vi "Read Fill.vi"(8 "error in (no error)":errorcluster, 11 "Rectangle in":refnum<class "Rectangle.lvclass">=refnum) -> (0 "error out":errorcluster, 2 "Fill":bool, 3 "Rectangle out":refnum<class "Rectangle.lvclass">)   [LabVIEW 2020]
uses:
  Rectangle.lvclass
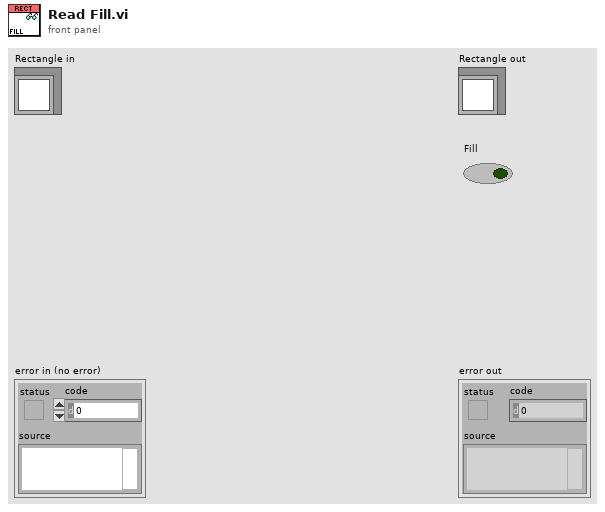
[diagram p1: front panel]
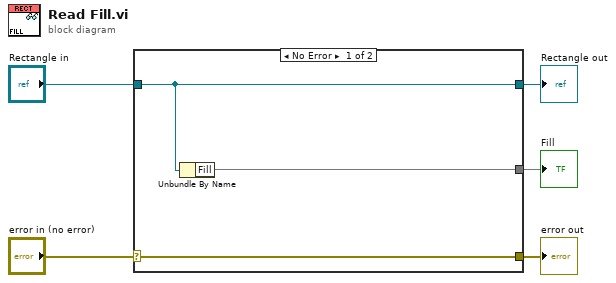
[diagram p0: block diagram]
diagram:
  n1 = case shown="No Error" "error in (no error)" {
    selector: "error in (no error)" -> [w8 w9]
    tunnel: [w8 w9] -> w4
    tunnel: [w7 w10] -> w2
    tunnel: "Rectangle in" -> [w7 w10]
    tunnel: [w6 _] -> w1
    frame No Error {
      n2 = Unbundle By Name(w7) -> ("Fill"=w6)
    }
    frame Error {
    }
  }
  "error out" <- w4
  "Rectangle out" <- w2
  "Fill" <- w1
